vi "shape detect work.vi"() -> ()   [LabVIEW 2016]
panel:
  out "d":dbl
  out "Image 2":T1(plugin-control)
  out "Particle Measurements (Pixels) (Particle Analysis 1)[0] 2":dbl
  out "Numeric 4":dbl
  out "Particle Measurements (Pixels) (Particle Analysis 1)[0]":dbl
  out "Centroid (pic center)":cluster{"X Centroid":sgl, "Y Centroid":sgl} {"Y Centroid" format="%.2f"; "X Centroid" format="%.2f"}
  out "Particle Measurements (Pixels) (Particle Analysis 1)":dbl[][](array[numeric]) format="%.2f"
  out "Number of Particles (Particle Analysis 1)":i32
  in  "Stop (F)":bool
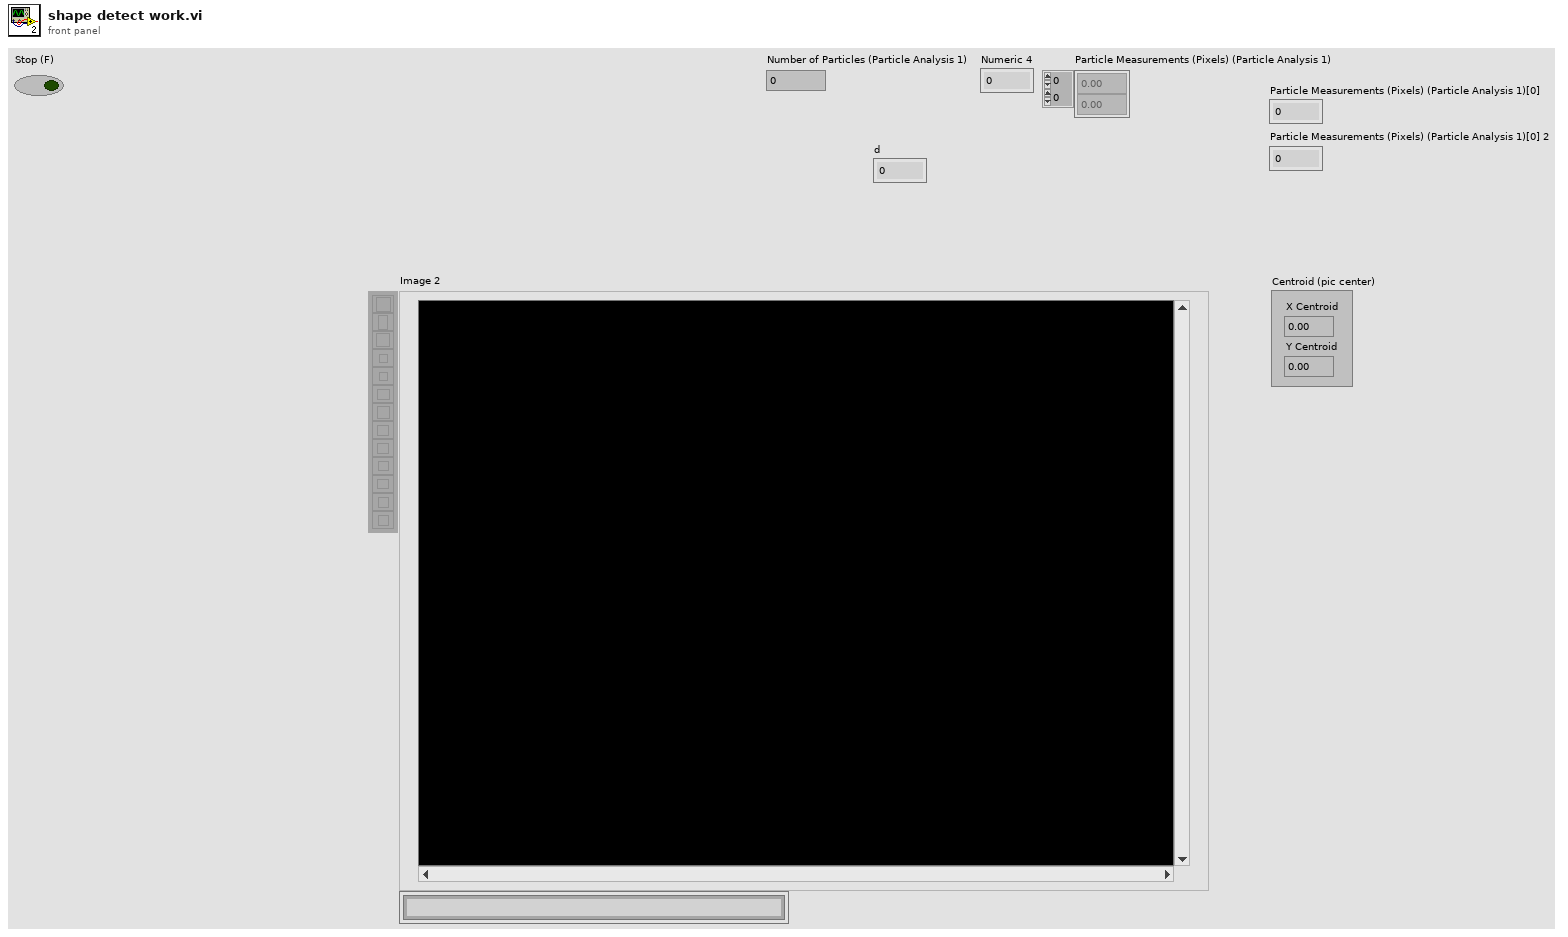
[diagram p1: front panel]
types:
  T1 = typedef "IMAQ Image.ctl" = refnum<image>
  T2 = typedef "Image Type" = u32
  T3 = cluster{"Particle Measurements (Pixels) (Particle Analysis 2)[0]":dbl, "Particle Measurements (Pixels) (Particle Analysis 2)[1]":dbl, "Particle Measurements (Pixels) (Particle Analysis 2)[2]":dbl, "Particle Measurements (Pixels) (Particle Analysis 2)[3]":dbl, "Particle Measurements (Pixels) (Particle Analysis 2)[4]":dbl, "Particle Measurements (Pixels) (Particle Analysis 2)[5]":dbl, "Particle Measurements (Pixels) (Particle Analysis 2)[6]":dbl, "Particle Measurements (Pixels) (Particle Analysis 2)[7]":dbl, "Particle Measurements (Pixels) (Particle Analysis 2)[8]":dbl}
  T4 = cluster{"Particle Measurements (Pixels) (Particle Analysis 1)[0]":dbl, "Particle Measurements (Pixels) (Particle Analysis 1)[1]":dbl, "Particle Measurements (Pixels) (Particle Analysis 1)[2]":dbl, "Particle Measurements (Pixels) (Particle Analysis 1)[3]":dbl, "Particle Measurements (Pixels) (Particle Analysis 1)[4]":dbl, "Particle Measurements (Pixels) (Particle Analysis 1)[5]":dbl, "Particle Measurements (Pixels) (Particle Analysis 1)[6]":dbl, "Particle Measurements (Pixels) (Particle Analysis 1)[7]":dbl, "Particle Measurements (Pixels) (Particle Analysis 1)[8]":dbl}
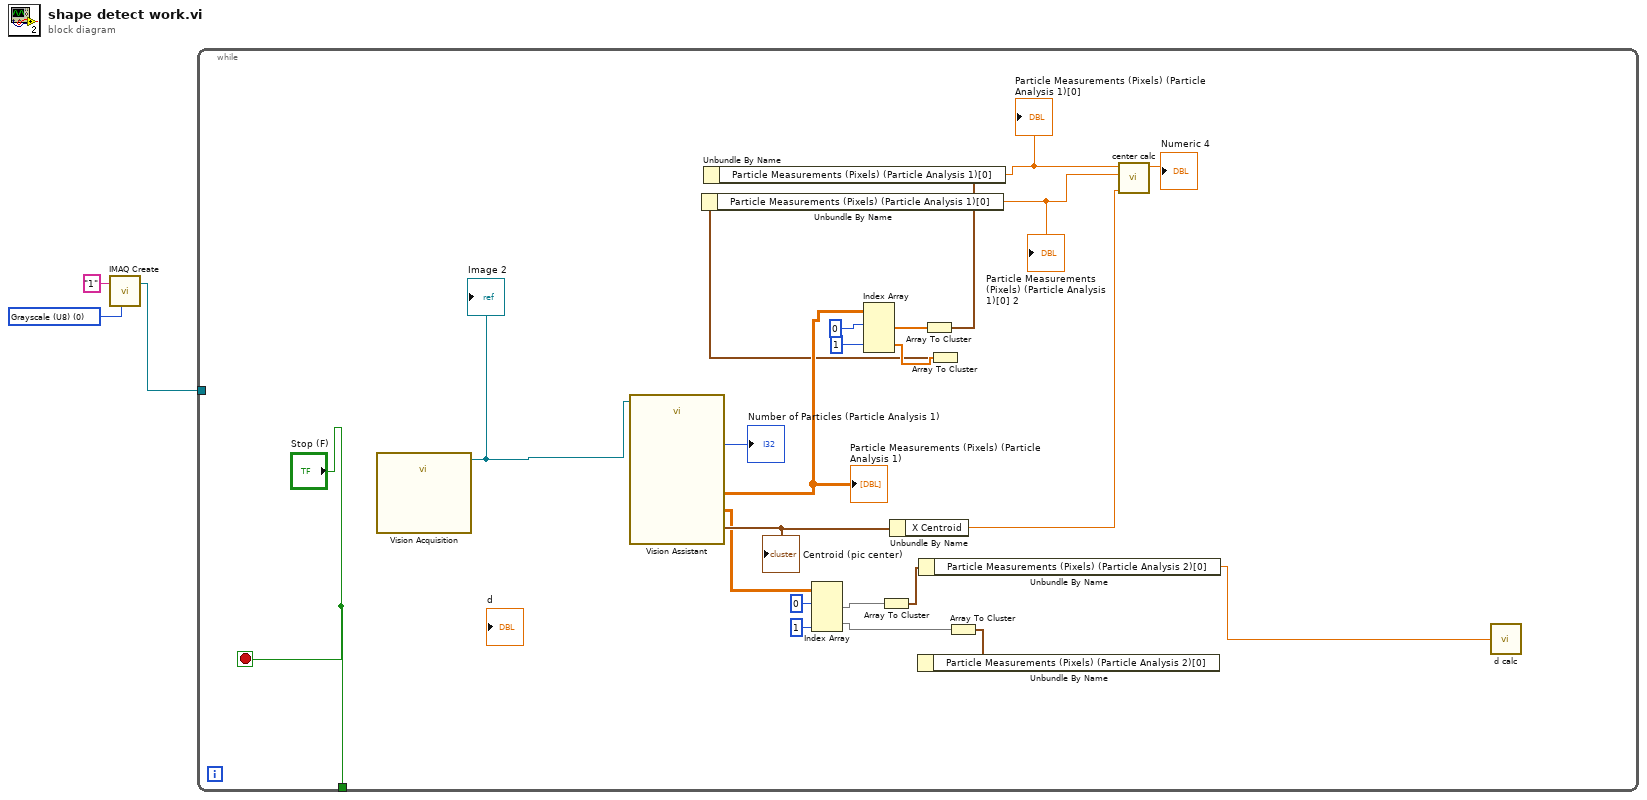
[diagram p0: block diagram]
diagram:
  w2 = T2 0 items=["Grayscale (U8)", "Grayscale (I16)", "Grayscale (SGL)", "Complex (CSG)", "RGB (U32)", "HSL (U32)", "RGB (U64)", "Grayscale (U16)"] ("Image Type")
  n1 = call "IMAQ Create"("Image Name"="1", "Image Type"=w2) -> ("New Image"=w1:T1)  [unwired: 3 in, 1 out]
  n2 = while {
    tunnel: ["Stop (F)"] -> _
    tunnel: w1 -> [_]
    stop <- "Stop (F)" stop-if-true
    n3 = call "Vision Acquisition"() -> ("Image Out"=w12:T1)  [unwired: 26 in, 1 out]
    "Image 2" <- w12
    n4 = call "Vision Assistant"("Image In"=w12) -> ("Number of Particles (Particle Analysis 1)"=→"Number of Particles (Particle Analysis 1)":i32, "Particle Measurements (Pixels) (Particle Analysis 1)"=w24:dbl[][], "Particle Measurements (Pixels) (Particle Analysis 2)"=w11:dbl[][], "Centroid (pic center)"=w20:cluster{"X Centroid":sgl, "Y Centroid":sgl})  [unwired: 21 in, 2 out]
    "Particle Measurements (Pixels) (Particle Analysis 1)" <- w24
    "Centroid (pic center)" <- w20
    n5 = Index Array(array=w11, index (row) #1=0 ("index (row)"), index (col) #2=1 ("disabled index (col)")) -> (element #1=w9:dbl[], element #2=w6:dbl[])  [unwired: 2 in]
    n6 = Index Array(array=w24, index (row) #1=0 ("index (row)"), index (row) #2=1 ("disabled index (row)")) -> (element #1=w23:dbl[], element #2=w16:dbl[])  [unwired: 2 in]
    n7 = Array To Cluster(array=w9) -> (cluster=w8:T3)
    n8 = Unbundle By Name(w20) -> ("X Centroid"=w19:sgl)
    n9 = Unbundle By Name(w8) -> ("Particle Measurements (Pixels) (Particle Analysis 2)[0]"=w4:dbl)
    n10 = Array To Cluster(array=w23) -> (cluster=w22:T4)
    n11 = Unbundle By Name(w22) -> ("Particle Measurements (Pixels) (Particle Analysis 1)[0]"=w21:dbl)
    "Particle Measurements (Pixels) (Particle Analysis 1)[0]" <- w21
    n12 = Array To Cluster(array=w16) -> (cluster=w15:T4)
    n13 = Unbundle By Name(w15) -> ("Particle Measurements (Pixels) (Particle Analysis 1)[0]"=w14:dbl)
    "Particle Measurements (Pixels) (Particle Analysis 1)[0] 2" <- w14
    n14 = Array To Cluster(array=w6) -> (cluster=w5:T3)
    n15 = Unbundle By Name(w5) -> ()  [unwired: 1 out]
    n16 = call "center calc.vi"("Numeric 3"=w19, 10:w14, 11:w21) -> ("Numeric 4"=→"Numeric 4":dbl)  [unwired: 8 in]
    n17 = call "d calc.vi"("y p"=w4) -> ()  [unwired: 7 in, 1 out]
  }
